vi "Server.vi"() -> ()   [LabVIEW 2018]
panel:
  out "length":i32
  in  "bytes to read":i32=100
  out "received message":string
  in  "stop":bool
  in  "listening port":u16=50001
  # "TCP Server"
  # "restart VI after changing\nlistening port number"
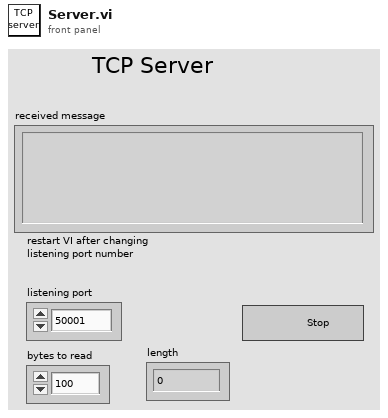
[diagram p1: front panel]
types:
  T1 = enum16{"Standard", "Buffered", "CRLF", "Immediate"}
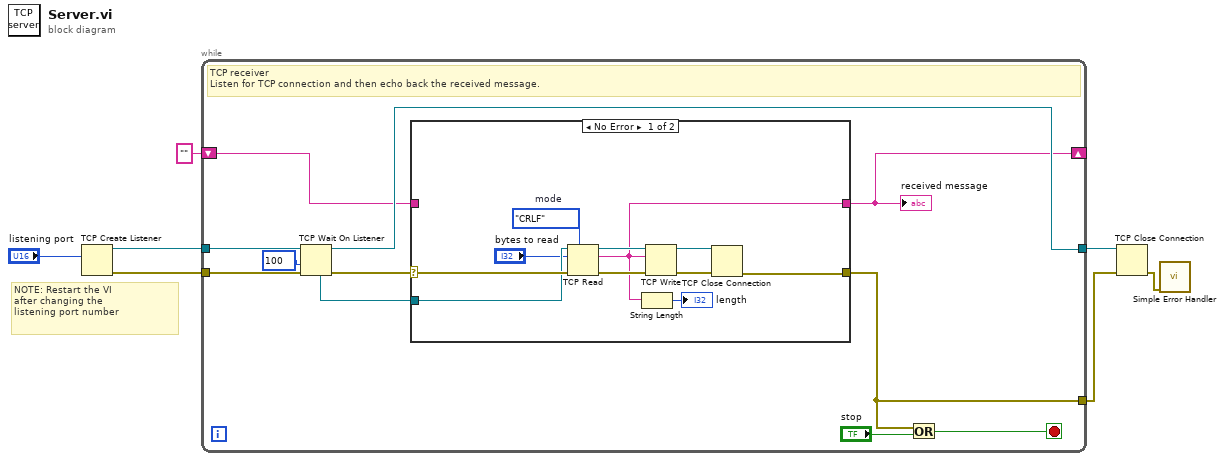
[diagram p0: block diagram]
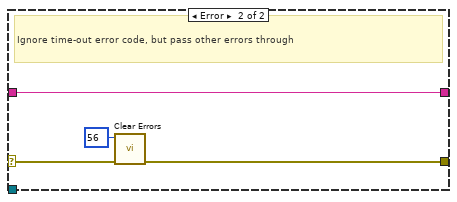
[diagram p2: hidden frame]
diagram:
  # "NOTE: Restart the VI\nafter changing the\nlistening port number"
  n1 = TCP Create Listener(10:"listening port") -> (0:w7:errorcluster, 3:w6:refnum<k5>)  [unwired: 4 in, 1 out]
  n2 = while {
    tunnel: w6 -> [w18]
    tunnel: [w14] -> w2
    tunnel: w7 -> [w17]
    tunnel: [w11] -> w4
    shift-right: [w8] -> _
    shift-left: "" ("data out") -> [w9]
    stop <- w12 stop-if-true
    # "TCP receiver\nListen for TCP connection and then echo back the received message."
    n3 = TCP Wait On Listener(8:w17, 9:100 ("timeout ms (25000)"), 11:w18) -> (0:w16:errorcluster, 3:w14:refnum<k5>, 4:w10:refnum<k5>)  [unwired: 1 in, 2 out]
    n4 = case shown="No Error" w16 {
      selector: w16 -> [w24 w33]
      tunnel: [w23 w32] -> w11
      tunnel: w10 -> [w22 _]
      tunnel: [w20 w30] -> w8
      tunnel: w9 -> [_ w30]
      frame No Error {
        w25 = T1."CRLF"  # mode
        n5 = TCP Read(connection ID=w22, bytes to read="bytes to read", error in (no error)=w24, 7:w25) -> (connection ID out=w27:refnum<k5>, data out=w20:string, error out=w29:errorcluster)  [unwired: 1 in]
        n6 = String Length(string=w20) -> (length=→"length":i32)
        n7 = TCP Write(connection ID=w27, data in=w20, error in (no error)=w29) -> (connection ID out=w28:refnum<k5>, error out=w26:errorcluster)  [unwired: 1 in, 1 out]
        n8 = TCP Close Connection(connection ID=w28, error in (no error)=w26) -> (error out=w23:errorcluster)  [unwired: 1 in, 1 out]
      }
      frame Error {
        # "Ignore time-out error code, but pass other errors through"
        n9 = call <vilib>:"Clear Errors.vi"("error in (no error)"=w33, "specific error code to clear (0: all)"=56) -> ("error out"=w32:errorcluster)  [unwired: 4 in, 1 out]
      }
    }
    "received message" <- w8
    n10 = Or(x=w11, y="stop") -> (x .or. y?=w12:bool)
  }
  n11 = TCP Close Connection(connection ID=w2, error in (no error)=w4) -> (error out=w5:errorcluster)  [unwired: 1 in, 1 out]
  n12 = call <vilib>:"Simple Error Handler.vi"("error in (no error)"=w5) -> ()  [unwired: 4 in, 5 out]
